vi "SeriellLesen.vi"(0 "VISA resource name":refnum<visa-resource-name>, 1 "error in (no error)":errorcluster) -> (2 "Temperatur":dbl, 3 "Humidity":dbl, 4 "VISA resource name 2":refnum<visa-resource-name>, 5 "error out":errorcluster)   [LabVIEW 2021]
panel:
  in  "stop":bool
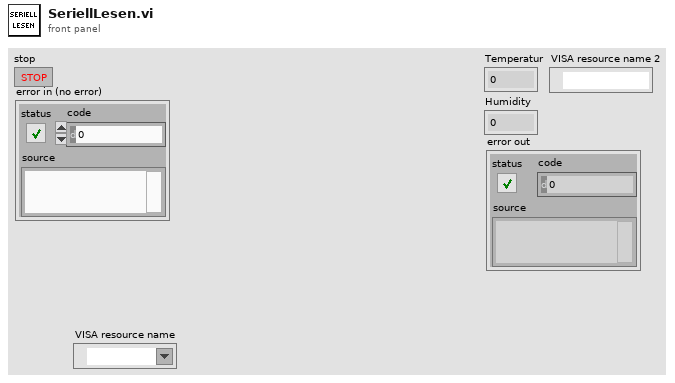
[diagram p1: front panel]
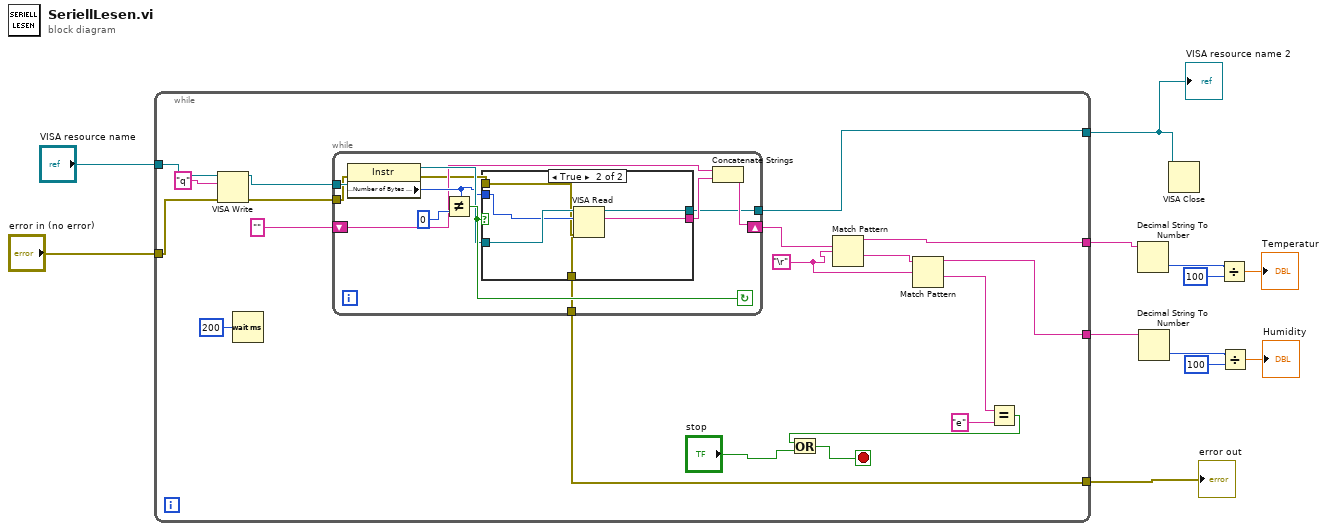
[diagram p0: block diagram]
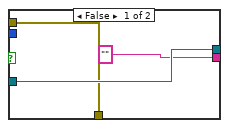
[diagram p2: hidden frame]
diagram:
  n1 = while {
    tunnel: "VISA resource name" -> [w31]
    tunnel: [w27] -> w11
    tunnel: [w21] -> w10
    tunnel: [w16] -> w3
    tunnel: "error in (no error)" -> [w15]
    tunnel: [w13] -> w1
    stop <- w22 stop-if-true
    w18 = "\r"
    n2 = VISA Write(VISA resource name=w31, write buffer="q", error in (no error)=w15) -> (VISA resource name out=w20:refnum<visa-resource-name>, error out=w14:errorcluster)  [unwired: 1 out]
    n3 = Wait (ms)(milliseconds to wait=u32 200) -> ()  [unwired: 1 out]
    n4 = while {
      tunnel: w20 -> [w43]
      shift-right: [w36] -> w26
      shift-left: "" -> [w37]
      tunnel: [w35] -> w27
      tunnel: w14 -> [w34]
      tunnel: [w32] -> w13
      stop <- w41 continue-if-true
      n5 = property class="Instr"(reference=w43, error in=w34) -> (reference out=w40:refnum<visa-resource-name>, error out=w33:errorcluster, "Serial Settings:Number of Bytes at Serial Port"=w39:u32)
      n6 = Not Equal?(x=w39, y=u32 0) -> (x != y?=w41:bool)
      n7 = case shown="True" w41 {
        tunnel: w40 -> [w46 w52]
        tunnel: w39 -> [_ w51]
        tunnel: ["" ("read buffer") w50] -> w38
        tunnel: [w46 w49] -> w35
        tunnel: w33 -> [w44 w48]
        tunnel: [w44 w47] -> w32
        frame False {
        }
        frame True {
          n8 = VISA Read(VISA resource name=w52, byte count=w51, error in (no error)=w48) -> (VISA resource name out=w49:refnum<visa-resource-name>, read buffer=w50:string, error out=w47:errorcluster)  [unwired: 1 out]
        }
      }
      n9 = Concatenate Strings(w37, w38) -> (w36:string)
    }
    n10 = Match Pattern(string=w26, regular expression=w18) -> (before substring=w21:string, after substring=w19:string)  [unwired: 1 in, 2 out]
    n11 = Match Pattern(string=w19, regular expression=w18) -> (before substring=w16:string, after substring=w17:string)  [unwired: 1 in, 2 out]
    n12 = Equal?(x=w17, y="e" ("string")) -> (x = y?=w23:bool)
    n13 = Or(x=w23, y="stop") -> (x .or. y?=w22:bool)
  }
  "error out" <- w1
  "VISA resource name 2" <- w11
  n14 = Decimal String To Number(string=w10) -> (number=w9:i32)  [unwired: 2 in, 1 out]
  n15 = Decimal String To Number(string=w3) -> (number=w6:i32)  [unwired: 2 in, 1 out]
  n16 = VISA Close(VISA resource name=w11) -> ()  [unwired: 1 in, 1 out]
  n17 = Divide(x=w9, y=100) -> (x/y=→"Temperatur":dbl)
  n18 = Divide(x=w6, y=100) -> (x/y=→"Humidity":dbl)
